vi "Display window.vi"(0 "Child Hwnd":u32, 11 "error in (no error)":errorcluster) -> (15 "error out":errorcluster)   [LabVIEW 2016, in "LV MDI.lvclass"]
doc: "Display the window for which handle is provided."
uses:
  LV MDI.lvclass
  user32.dll
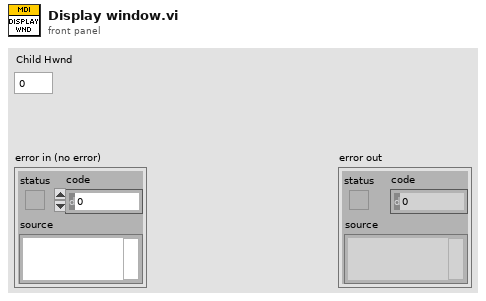
[diagram p1: front panel]
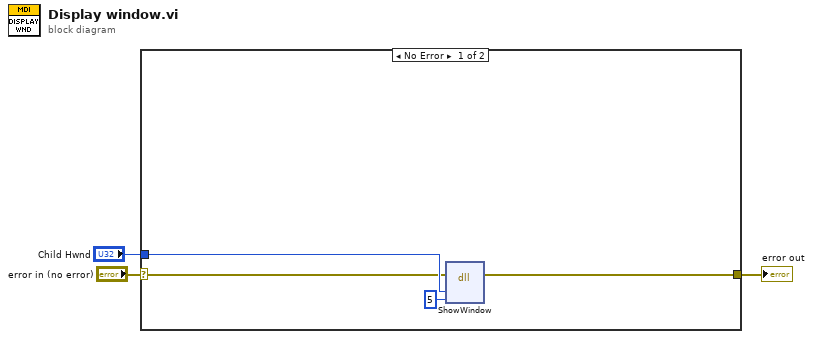
[diagram p0: block diagram]
diagram:
  n1 = case shown="No Error" "error in (no error)" {
    selector: "error in (no error)" -> [w4 w8]
    tunnel: [w6 w8] -> w2
    tunnel: "Child Hwnd" -> [w5 _]
    frame No Error {
      n2 = dll-call lib="user32.dll" fn="ShowWindow"(error in=w4, "hwnd"=w5, "nCmdShow"=u32 5) -> (error out=w6:errorcluster)  [unwired: 5 in, 1 out]
    }
    frame Error {
    }
  }
  "error out" <- w2
